vi "Initialize.vi"(8 "error in (no error)":errorcluster, 9 "Requestor":string, 10 "Requestee":string, 11 "Meter Measurement in":refnum<class "Meter Measurement.lvclass">) -> (0 "error out":errorcluster, 3 "Meter Measurement out":refnum<class "Meter Measurement.lvclass">)   [LabVIEW 2015, in "Meter Measurement.lvclass"]
uses:
  Meter Measurement.lvclass
  Mag Lab Root/Mag Lab Root.lvclass/Mag Lab Root.ctl
  <vilib>/ActorFramework/Actor/Actor.lvclass/Actor.ctl
  Meter Measurement.lvclass/Meter Measurement.ctl
  Mag Lab Root Messages/Initialize Msg/Initialize Msg.lvclass/Initialize Msg.ctl
  <vilib>/ActorFramework/Message Enqueuer/Message Enqueuer.lvclass/Message Enqueuer.ctl
  <vilib>/ActorFramework/Message Enqueuer/Enqueue.vi
  <vilib>/ActorFramework/Message Priority Queue/Priority Enqueue.vi
  Mag Lab Root Messages/Initialize Msg/Initialize Msg.lvclass
  <vilib>/ActorFramework/Actor/Actor.lvclass
  Mag Lab Root/Mag Lab Root.lvclass
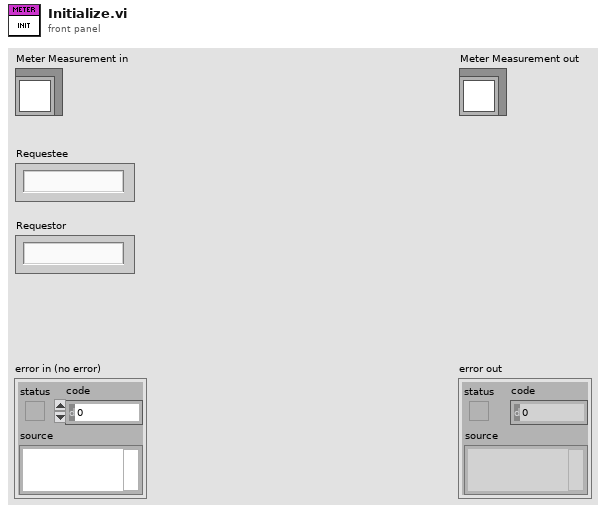
[diagram p1: front panel]
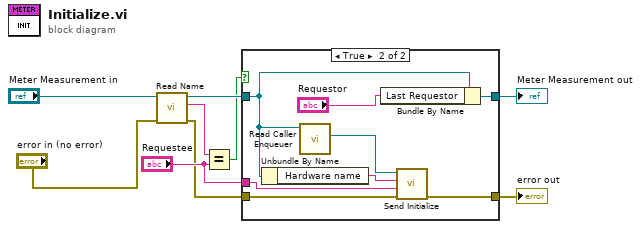
[diagram p0: block diagram]
diagram:
  n1 = call "Read Name.vi"("error in (no error)"="error in (no error)", "Mag Lab Root in"="Meter Measurement in") -> ("error out"=w1:errorcluster, "Name"=w6:string, "Mag Lab Root out"=w7:refnum<class "Meter Measurement.lvclass">)  [unwired: 7 in]
  n2 = Equal?(x=w6, y="Requestee") -> (x = y?=w4:bool)
  n3 = case shown="True" w4 {
    tunnel: w1 -> [w10 w18]
    tunnel: [w10 w17] -> w9
    tunnel: w7 -> [w11 w14]
    tunnel: "Requestee" -> [_ w16]
    tunnel: [w11 w12] -> w3
    frame False {
    }
    frame True {
      n4 = Unbundle By Name(w14) -> ("Hardware name"=w15:string)
      n5 = call <vilib>:"Read Caller Enqueuer.vi"("Actor"=w14) -> ("Caller Enqueuer"=w19:refnum<class "Message Enqueuer.lvclass">)  [unwired: 10 in]
      n6 = Bundle By Name(cluster=w14, "Last Requestor"="Requestor") -> (w12:refnum<class "Meter Measurement.lvclass">)
      n7 = call "Send Initialize.vi"("error in (no error)"=w18, "Requestor"=w16, "Requestee"=w15, "Message Enqueuer"=w19) -> ("error out"=w17:errorcluster)  [unwired: 6 in, 1 out]
    }
  }
  "error out" <- w9
  "Meter Measurement out" <- w3
